vi "RSZVB Set Dummy Source Power Calibration State.vi"(7 "Dummy Source Power Calibration (F: Off)":bool, 8 "error in (no error)":errorcluster {"code" format="%.0x"}, 9 "Port Number (1)":i32=1, 10 "Channel (1)":i32=1, 11 "VISA session":refnum<visa-resource-name>) -> (0 "error out":errorcluster {"code" format="%.0x"}, 3 "dup VISA session":refnum<visa-resource-name>)   [LabVIEW 2011]
doc: "This VI enables the analyzer to create a set of default source power calibration data. The analyzer uses the reference channel power to acquire the default calibration data. No external power meter is required. \n\nNotes:\n\n(1) The main purpose of the default calibration data set is to provide a dummy power calibration which you can replace with your own, external power calibration data. You may have acquired the external data in a previous session or even on an other instrument. If you want to use the external power calibration data on the analyzer, generate the default data set first and overwrite it with the external data.\n\nRemote-control command(s):\nSOURce<Ch>:POWer<Pt>:CORRection:DEFault ON | OFF"
uses:
  _utility/RSZVB Global Data.vi
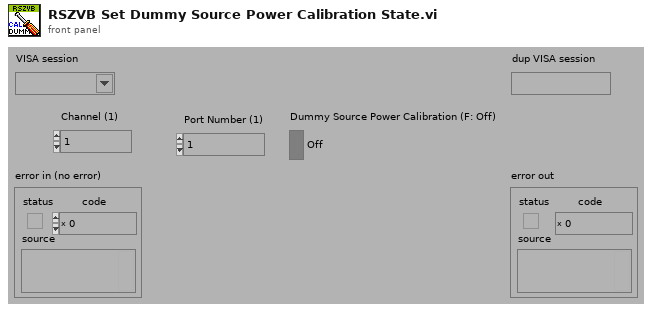
[diagram p1: front panel]
types:
  T1 = cluster{"Error Checking (T: On)":bool, "Installed Options":string[], "Data Valid?":bool, "Ports":i32, "Model":string[], "Option Checking (T: On)":bool}[]
  T2 = cluster{"Error Checking (T: On)":bool, "Installed Options":string[], "Data Valid?":bool, "Ports":i32, "Model":string[], "Option Checking (T: On)":bool}
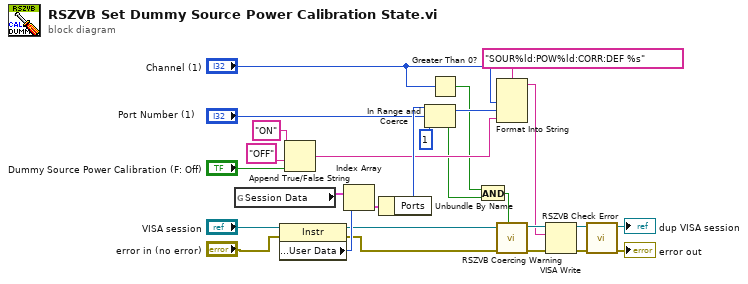
[diagram p0: block diagram]
diagram:
  n1 = global read "RSZVB Global Data.vi" "Session Data"() -> (w21:T1)
  n2 = property class="Instr"(reference="VISA session", error in="error in (no error)") -> (reference out=w19:refnum<visa-resource-name>, error out=w1:errorcluster, "General Settings:User Data"=w22:u32)
  n3 = Append True/False String(1:"Dummy Source Power Calibration (F: Off)", 2:"OFF" ("false string"), 3:"ON" ("true string")) -> (0:w11:string)  [unwired: 1 in]
  n4 = Index Array(array=w21, index=w22) -> (element=w20:T2)
  n5 = Unbundle By Name(w20) -> ("Ports"=w15:i32)
  n6 = In Range and Coerce(upper limit=w15, x="Port Number (1)", lower limit=1) -> (coerced(x)=w12:i32, In Range?=w5:bool)
  n7 = Greater Than 0?(x="Channel (1)") -> (x > 0?=w4:bool)
  n8 = And(x=w4, y=w5) -> (x .and. y?=w10:bool)
  n9 = Format Into String(format string="SOUR%ld:POW%ld:CORR:DEF %s", "Channel (1)", w12, w11) -> (resulting string=w3:string)  [unwired: 2 in, 1 out]
  n10 = call "RSZVB Coercing Warning.vi"("In Range?"=w10, "error in (no error)"=w1, "VISA session"=w19) -> ("error out"=w25:errorcluster, "dup VISA session"=w8:refnum<visa-resource-name>)  [unwired: 7 in]
  n11 = VISA Write(VISA resource name=w8, write buffer=w3, error in (no error)=w25) -> (VISA resource name out=w7:refnum<visa-resource-name>, error out=w24:errorcluster)  [unwired: 1 out]
  n12 = call "RSZVB Check Error.vi"("error in (no error)"=w24, "VISA session"=w7) -> ("error out"=→"error out":errorcluster, "dup VISA session"=→"dup VISA session":refnum<visa-resource-name>)  [unwired: 8 in]
